vi "destoryChildEvents.vi"(8 "error in (no error)":errorcluster, 11 "cameraSettingsEventManager in":refnum<class "cameraSettingsEventManager.lvclass">) -> (0 "error out":errorcluster, 3 "cameraSettingsEventManager out":refnum<class "cameraSettingsEventManager.lvclass">)   [LabVIEW 2011, in "Tools.lvlib" / "Settings.lvlib" / "cameraSettingsEventManager.lvclass"]
uses:
  cameraSettingsEventManager.lvclass
  Tools/Settings.lvlib
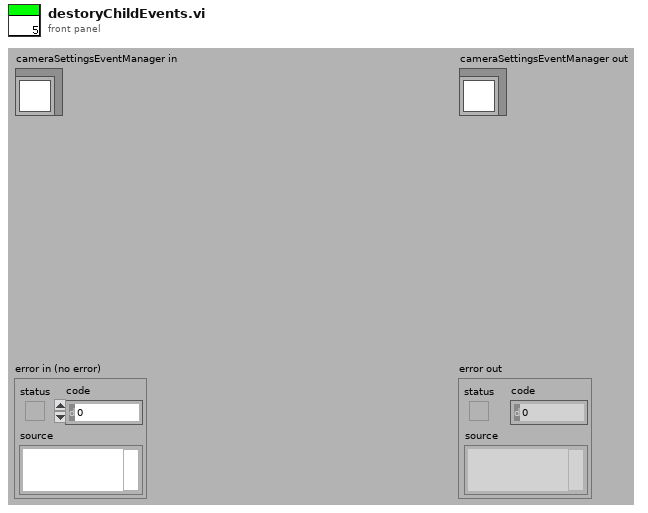
[diagram p1: front panel]
types:
  T1 = cluster{"loadCameraSettingsEvent":refnum<user-event>}
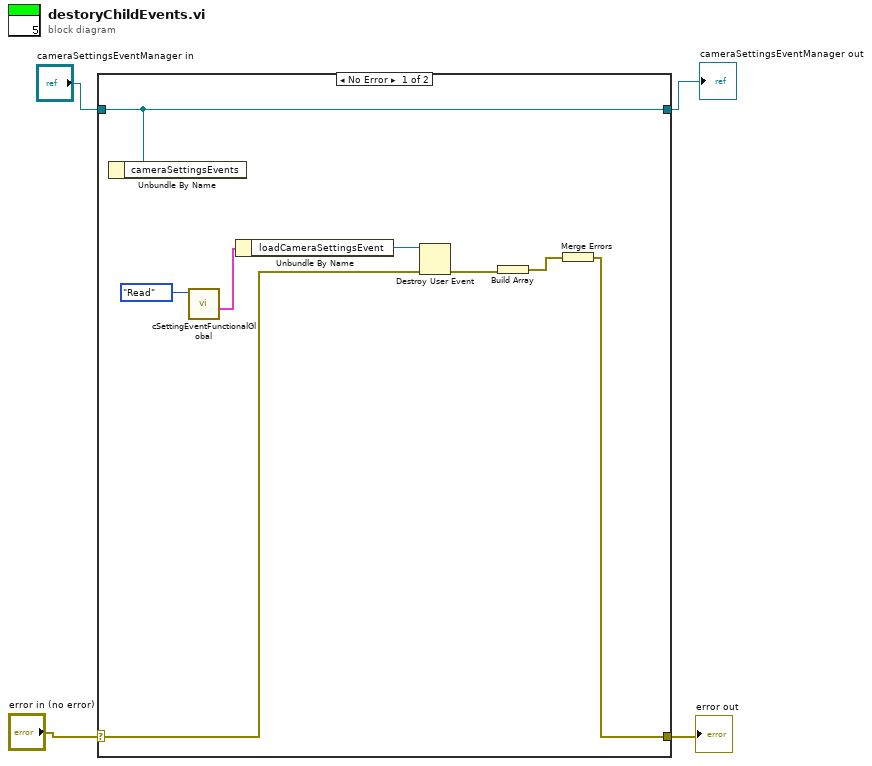
[diagram p0: block diagram]
diagram:
  n1 = case shown="No Error" "error in (no error)" {
    selector: "error in (no error)" -> [w9 w13]
    tunnel: [w6 w13] -> w3
    tunnel: "cameraSettingsEventManager in" -> [w5 w14]
    tunnel: [w5 w14] -> w1
    frame No Error {
      n2 = Unbundle By Name(w5) -> ()  [unwired: 1 out]
      n3 = call "cSettingEventFunctionalGlobal.vi"("Action"=enum16{"Write", "Read"}."Read") -> ("cameraSettingsEventsRef"=w11:T1)  [unwired: 10 in]
      n4 = Unbundle By Name(w11) -> ("loadCameraSettingsEvent"=w10:refnum<user-event>)
      n5 = Destroy User Event(user event=w10, error in=w9) -> (error out=w8:errorcluster)
      n6 = Build Array(w8) -> (w7:errorcluster[])
      n7 = Merge Errors(w7) -> (w6:errorcluster)
    }
    frame Error {
    }
  }
  "error out" <- w3
  "cameraSettingsEventManager out" <- w1
